vi "Custom Debug Data.vi"(0 "subroutine":string, 11 "error in":errorcluster) -> (4 "debug info":string, 15 "error out":errorcluster)   [LabVIEW 2021, in "Event Logger.lvlib"]
uses:
  Event Logger.lvlib
  <vilib>/Utility/error.llb/DialogType.ctl
  Converter/Converter Reusables/Converter Reusables.lvlib
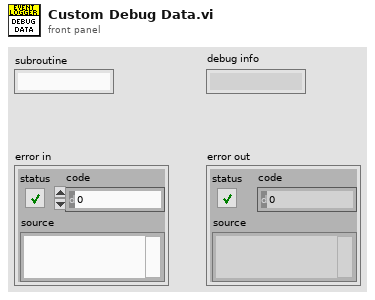
[diagram p1: front panel]
types:
  T1 = typedef "DialogType.ctl" = u16
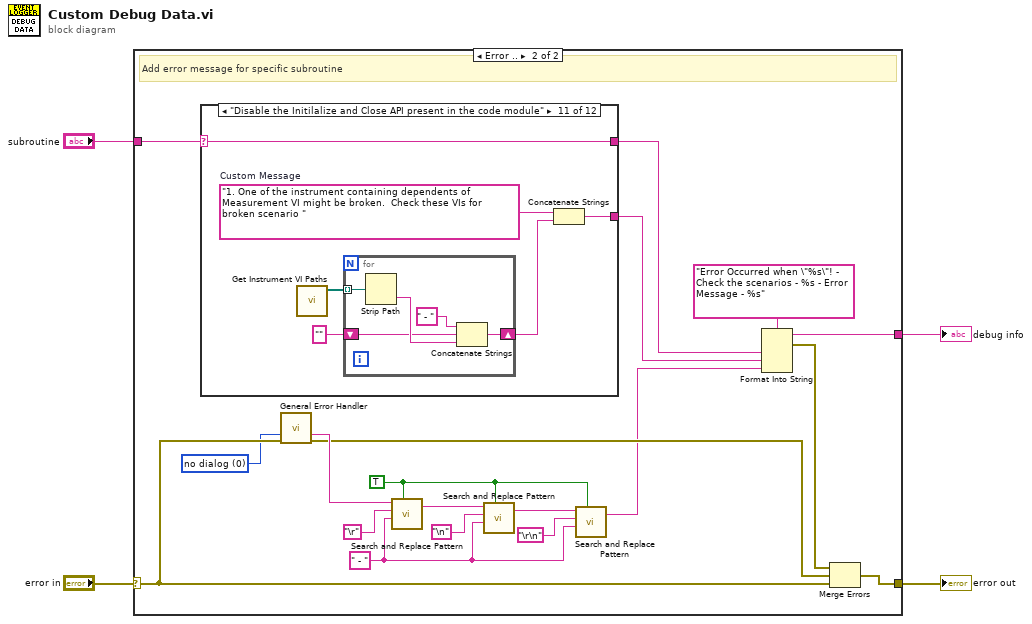
[diagram p0: block diagram]
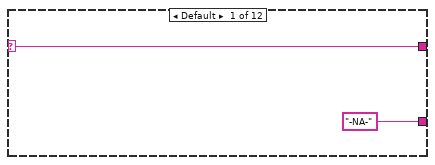
[diagram p3: hidden frame]
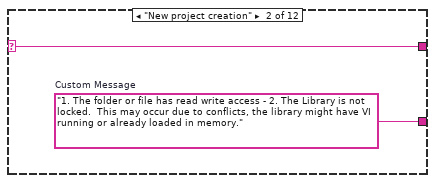
[diagram p4: hidden frame]
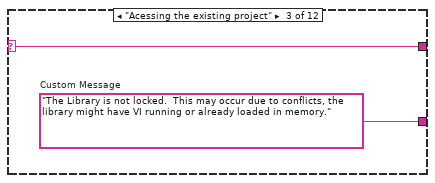
[diagram p5: hidden frame]
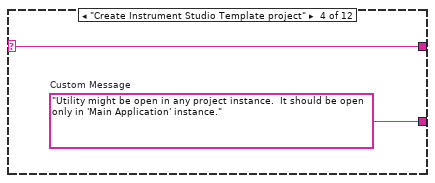
[diagram p6: hidden frame]
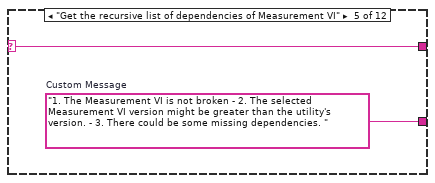
[diagram p7: hidden frame]
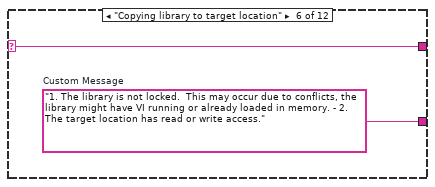
[diagram p8: hidden frame]
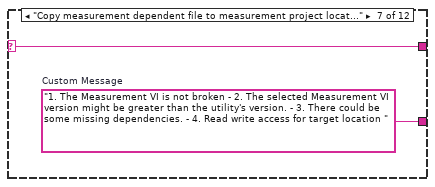
[diagram p9: hidden frame]
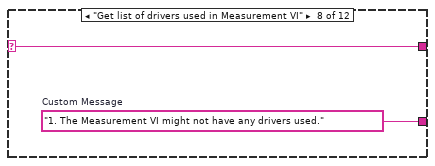
[diagram p10: hidden frame]
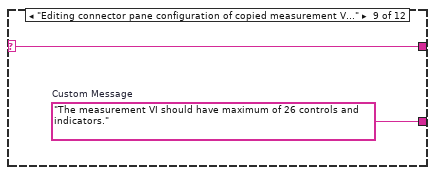
[diagram p11: hidden frame]
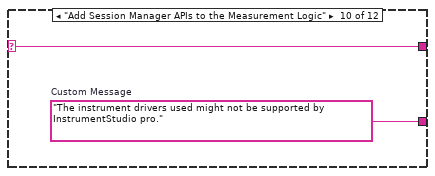
[diagram p12: hidden frame]
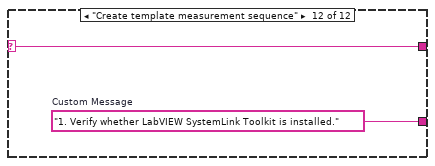
[diagram p13: hidden frame]
diagram:
  n1 = case shown="Error .." "error in" {
    selector: "error in" -> [w5 w23]
    tunnel: [w5 w24] -> w4
    tunnel: "subroutine" -> [_ w8]
    tunnel: [_ w10] -> w1
    frame No Error {
    }
    frame Error {
      w14 = TRUE ("replace all? (F)")
      w21 = " - "
      w22 = T1 0 items=["no dialog", "OK message", "continue or stop message", "OK message + warnings", "continue/stop + warnings"] ("type of dialog (OK msg:1)")
      # "Add error message for specific subroutine"
      n2 = case shown="\"Disable the Initilalize and Close API present in the code module\"" w8 {
        selector: w8 -> [w25 w27 w29 w31 w33 w35 w37 w39 w41 w43 w45 w56]
        tunnel: ["-NA-" ("Custom Message") w28 w30 w32 w34 w36 w38 w40 w42 w44 w47 w57] -> w6
        tunnel: [w25 w27 w29 w31 w33 w35 w37 w39 w41 w43 w45 w56] -> w7
        frame Default {
        }
        frame "New project creation" {
          w28 = "1. The folder or file has read write access - 2. The Library is not locked.  This may occur due to conflicts, the library might have VI running or already loaded in memory."  # Custom Message
        }
        frame "Acessing the existing project" {
          w30 = "The Library is not locked.  This may occur due to conflicts, the library might have VI running or already loaded in memory."  # Custom Message
        }
        frame "Create Instrument Studio Template project" {
          w32 = "Utility might be open in any project instance.  It should be open only in 'Main Application' instance."  # Custom Message
        }
        frame "Get the recursive list of dependencies of Measurement VI" {
          w34 = "1. The Measurement VI is not broken - 2. The selected Measurement VI version might be greater than the utility's version. - 3. There could be some missing dependencies. "  # Custom Message
        }
        frame "Copying library to target location" {
          w36 = "1. The library is not locked.  This may occur due to conflicts, the library might have VI running or already loaded in memory. - 2. The target location has read or write access."  # Custom Message
        }
        frame "Copy measurement dependent file to measurement project location" {
          w38 = "1. The Measurement VI is not broken - 2. The selected Measurement VI version might be greater than the utility's version. - 3. There could be some missing dependencies. - 4. Read write access for target location "  # Custom Message
        }
        frame "Get list of drivers used in Measurement VI" {
          w40 = "1. The Measurement VI might not have any drivers used."  # Custom Message
        }
        frame "Editing connector pane configuration of copied measurement VI" {
          w42 = "The measurement VI should have maximum of 26 controls and indicators."  # Custom Message
        }
        frame "Add Session Manager APIs to the Measurement Logic" {
          w44 = "The instrument drivers used might not be supported by InstrumentStudio pro."  # Custom Message
        }
        frame "Disable the Initilalize and Close API present in the code module" {
          w49 = "1. One of the instrument containing dependents of Measurement VI might be broken.  Check these VIs for broken scenario "  # Custom Message
          n3 = call "Get Instrument VI Paths.vi"() -> ("Instr VI Paths[]"=w48:path[])  [unwired: 10 in, 1 out]
          n4 = for {
            tunnel: w48 -> [w55] mode=indexing
            shift-right: [w51] -> w50
            shift-left: "" -> [w53]
            n5 = Strip Path(path=w55) -> (name=w54:string)  [unwired: 1 out]
            n6 = Concatenate Strings(" - " ("string"), w53, w54) -> (w51:string)
          }
          n7 = Concatenate Strings(w49, w50) -> (w47:string)
        }
        frame "Create template measurement sequence" {
          w57 = "1. Verify whether LabVIEW SystemLink Toolkit is installed."  # Custom Message
        }
      }
      n8 = call <vilib>:"General Error Handler.vi"("type of dialog (OK msg:1)"=w22, "error in (no error)"=w23) -> ("message"=w15:string, "error out"=w13:errorcluster)  [unwired: 9 in, 3 out]
      n9 = call <vilib>:"Search and Replace Pattern.vi"("string"=w15, "regular expression (\"\")"="\r", "replace string (\"\")"=w21, "replace all? (F)"=w14) -> ("result string"=w19:string)  [unwired: 1 in, 1 out]
      n10 = call <vilib>:"Search and Replace Pattern.vi"("string"=w19, "regular expression (\"\")"="\n", "replace string (\"\")"=w21, "replace all? (F)"=w14) -> ("result string"=w20:string)  [unwired: 1 in, 1 out]
      n11 = call <vilib>:"Search and Replace Pattern.vi"("string"=w20, "regular expression (\"\")"="\r\n", "replace string (\"\")"=w21, "replace all? (F)"=w14) -> ("result string"=w12:string)  [unwired: 1 in, 1 out]
      n12 = Format Into String(format string="Error Occurred when \"%s\"! - Check the scenarios - %s - Error Message - %s" ("Custom Message"), w7, w6, w12) -> (resulting string=w10:string, error out=w11:errorcluster)  [unwired: 2 in]
      n13 = Merge Errors(w11, w13, w23) -> (w24:errorcluster)
    }
  }
  "error out" <- w4
  "debug info" <- w1
